vi "Read Conpane Image.vi"(8 "error in (no error)":errorcluster, 11 "Vi in":refnum<class "Vi.lvclass">) -> (0 "error out":errorcluster, 2 "image data":T1, 3 "Vi out":refnum<class "Vi.lvclass">)   [LabVIEW 2021, in "TAF Proj Document Type.lvlib" / "Vi.lvclass"]
uses:
  <vilib>/Wovalab/AntiDoc/Document Type/Add-ons/LabVIEW TAF Project/Vi/Vi.lvclass
  <vilib>/picture/picture.llb/imagedata.ctl
  <vilib>/Wovalab/AntiDoc/Document Type/Add-ons/LabVIEW TAF Project/Vi/Vi.lvclass/Vi.ctl
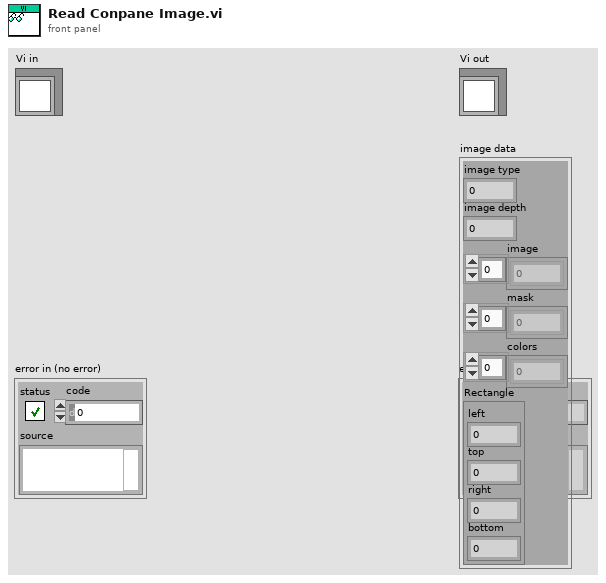
[diagram p1: front panel]
types:
  T1 = typedef "imagedata.ctl" = cluster{"image type":i32, "image depth":i32, "image":u8[], "mask":u8[], "colors":u32[], "Rectangle":cluster{"left":i16, "top":i16, "right":i16, "bottom":i16}}
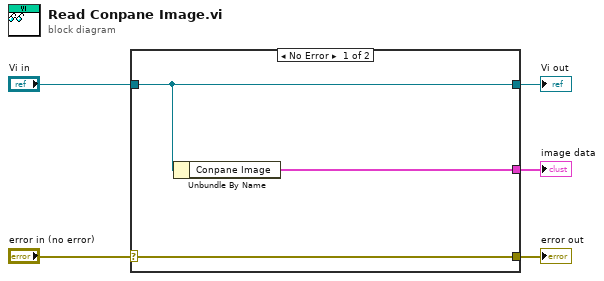
[diagram p0: block diagram]
diagram:
  n1 = case shown="No Error" "error in (no error)" {
    selector: "error in (no error)" -> [w8 w9]
    tunnel: [w8 w9] -> w4
    tunnel: [w7 w10] -> w2
    tunnel: "Vi in" -> [w7 w10]
    tunnel: [w6 _] -> w1
    frame No Error {
      n2 = Unbundle By Name(w7) -> ("Conpane Image"=w6:T1)
    }
    frame Error {
    }
  }
  "error out" <- w4
  "Vi out" <- w2
  "image data" <- w1
